vi "TestUplink.vi"(0 "RFSA Handle In":refnum<k15>="PXI1Slot5" caption="RFSA Handle in", 1 "UL Rx Span":i64=200000, 2 "SMU Handle In":refnum<k15> caption="SMU Handle in", 3 "UL Tx Payload (Hex)":string, 4 "UL Data Rate":i64=600, 5 "Resp Timeout (ms)":i32, 6 "FPGA Reference":refnum<k20>, 7 "error in (no error)":errorcluster, 8 "UL Freq Offset (Hz)":i64=1, 9 "UL Pwr Reduction (dB/2)":i8=-34, 10 "DxSupply":string, 11 "UL Tx Freq (Hz)":i64=1, 13 "UL Rx Timeout":i64=60, 14 "Enum":T1, 15 "UL Rx Central Freq":i64=902200000) -> (12 "Send UL OK":bool, 21 "Meas UL Rx Freq":i64, 23 "UL Rx Payload":string, 24 "Meas UL Idd":dbl, 27 "error out":errorcluster)   [LabVIEW 2018]
uses:
  Resources_Test/UART/ControlTestSlot.ctl
  <vilib>/Analysis/4window.llb/windowTd.ctl
  <vilib>/measure/maspectr.llb/FFT Power Spectrum and PSD for 1 Chan (CDB).vi
  <vilib>/measure/NI_MAPro.lvlib
  <vilib>/Analysis/NI_AALPro.lvlib
panel:
  out "Timeout Flag":bool
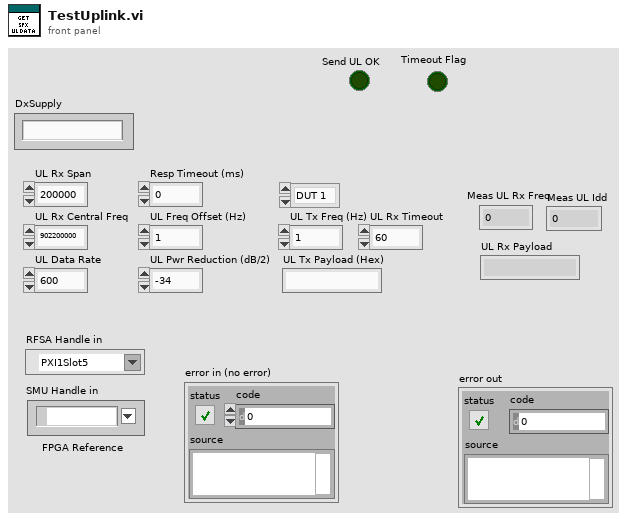
[diagram p1: front panel]
types:
  T1 = typedef "ControlTestSlot.ctl" = enum16{"DUT 1", "DUT 2"}
  T2 = cluster{"averaging mode":enum16{"No averaging", "Vector averaging", "RMS averaging", "Peak hold"}, "weighting mode":enum16{"Linear", "Exponential"}, "number of averages":u32}
  T3 = typedef "NI_AALPro.lvlib/windowTd.ctl" = u32
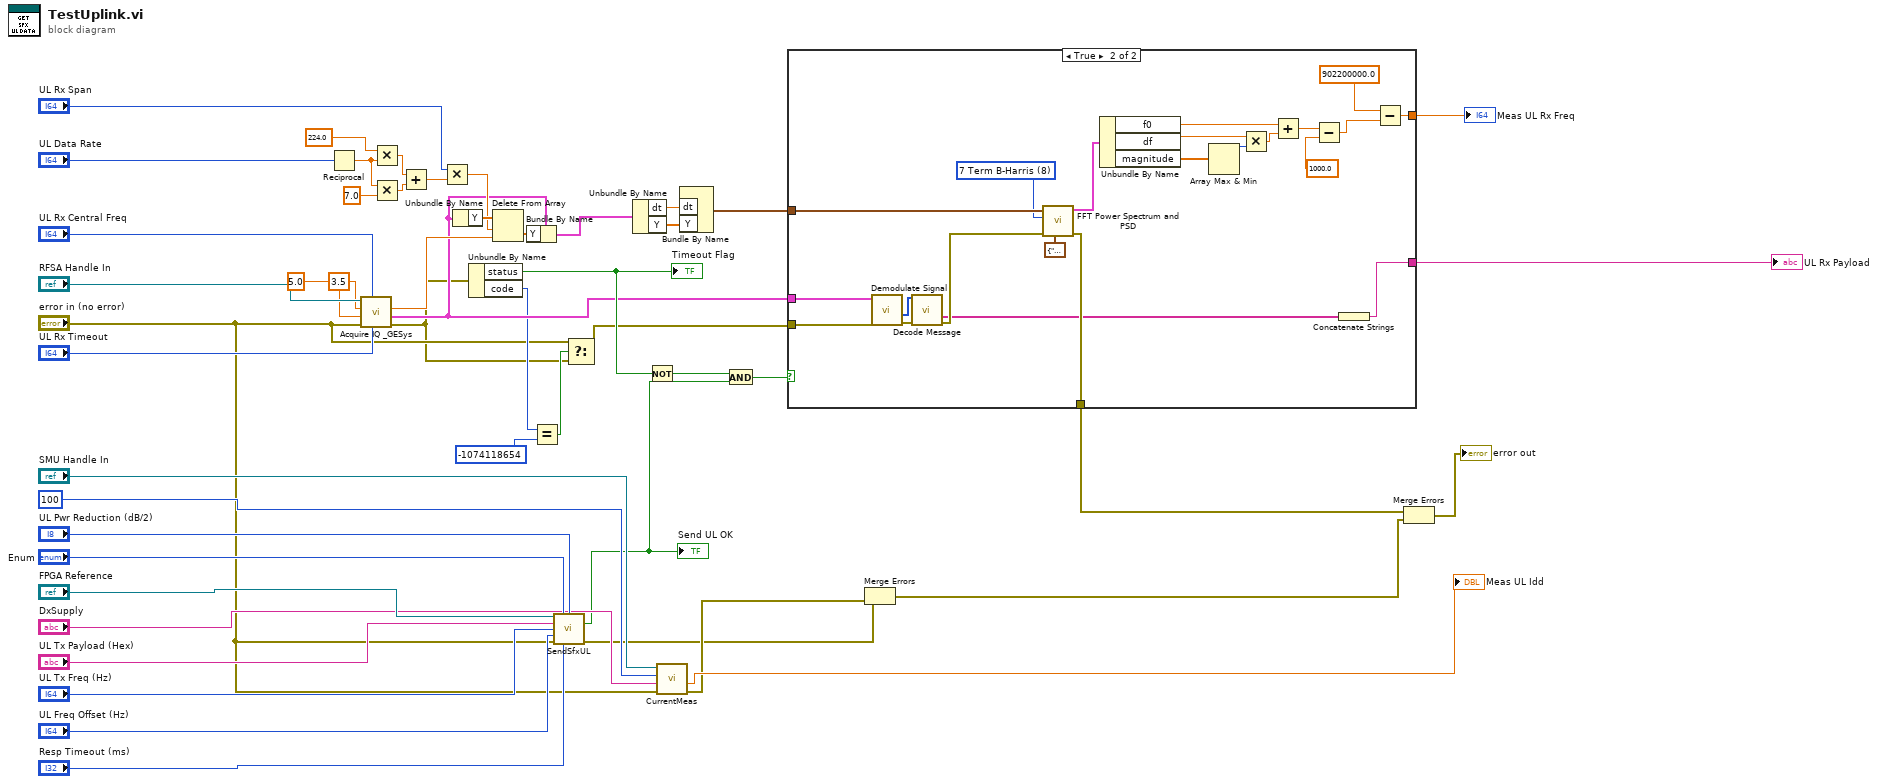
[diagram p0: block diagram]
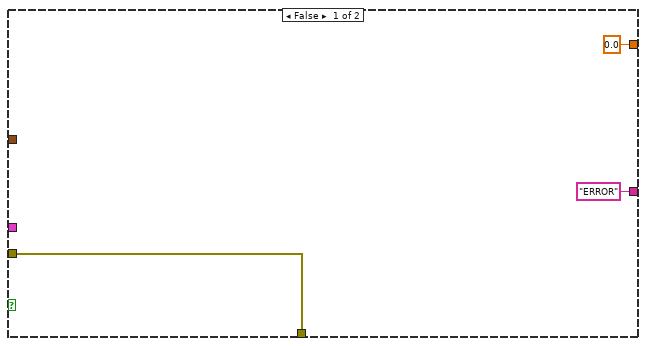
[diagram p2: hidden frame]
diagram:
  n1 = Reciprocal(x="UL Data Rate") -> (1/x=w27:dbl)
  n2 = call "Acquire IQ _GESys.vi"("timeout (10 sec)"="UL Rx Timeout", "Carrier Frequency (Hz)"="UL Rx Central Freq", "error in (no error)"="error in (no error)", "Reference Position (%)"=5.0, "Burst Length (sec)"=3.5, "instrument handle"="RFSA Handle In") -> ("error out"=w2:errorcluster, "IQ"=w8:cluster{"t0":dbl, "dt":dbl, "Y":cdb[]}, "Pre-Trigger"=w21:dbl)  [unwired: 2 in, 1 out]
  n3 = Multiply(x=224.0, y=w27) -> (x*y=w24:dbl)
  n4 = Multiply(x=w27, y=7.0) -> (x*y=w23:dbl)
  n5 = Add(x=w24, y=w23) -> (x+y=w25:dbl)
  n6 = Multiply(x="UL Rx Span", y=w25) -> (x*y=w22:dbl)
  n7 = Unbundle By Name(w8) -> ("Y"=w29:cdb[])
  n8 = Unbundle By Name(w2) -> ("status"=w15:bool, "code"=w6:i32)
  "Timeout Flag" <- w15
  n9 = Delete From Array(array=w29, length=w22, index=w21) -> (deleted portion=w20:cdb[])  [unwired: 1 out]
  n10 = Bundle By Name(cluster=w8, "Y"=w20) -> (w16:cluster{"t0":dbl, "dt":dbl, "Y":cdb[]})
  n11 = Equal?(x=w6, y=-1074118654) -> (x = y?=w4:bool)
  n12 = call "SendSfxUL.vi"("FPGA Reference"="FPGA Reference", "Enum"="Enum", "Pwr Reduction (dB/2)"="UL Pwr Reduction (dB/2)", "Tx Payload (Hex)"="UL Tx Payload (Hex)", "Tx Freq (Hz)"="UL Tx Freq (Hz)", "Freq Offset (Hz)"="UL Freq Offset (Hz)", "Error In"="error in (no error)", "Resp Timeout (ms)"="Resp Timeout (ms)") -> ("Send UL OK"=w13:bool, "Error Out"=w30:errorcluster)  [unwired: 6 in]
  "Send UL OK" <- w13
  n13 = Select(t="error in (no error)", s=w4, f=w2) -> (s? t:f=w1:errorcluster)
  n14 = Unbundle By Name(w16) -> ("dt"=w19:dbl, "Y"=w18:cdb[])
  n15 = Not(x=w15) -> (.not. x?=w14:bool)
  n16 = call "CurrentMeas.vi"("error in (no error)"="error in (no error)", "DxSupply"="DxSupply", "Measure Record Length"=100, "instrument handle"="SMU Handle In") -> ("error out"=w31:errorcluster, "Idd Peak"=→"Meas UL Idd":dbl)  [unwired: 4 in, 2 out]
  n17 = Bundle By Name("dt"=w19, "Y"=w18) -> (w17:waveform(cdb))  [unwired: 1 in]
  n18 = And(x=w14, y=w13) -> (x .and. y?=w9:bool)
  n19 = case shown="True" w9 {
    tunnel: [0.0 w75] -> w36
    tunnel: w17 -> [_ w74]
    tunnel: [w51 w61] -> w12
    tunnel: w1 -> [w51 w60]
    tunnel: w8 -> [_ w59]
    tunnel: ["ERROR" w54] -> w7
    frame False {
    }
    frame True {
      w66 = T3 8 items=["Rectangle"=0, "Hanning"=1, "Hamming"=2, "Blackman-Harris"=3, "Exact Blackman"=4, "Blackman"=5, "Flat Top"=6, "4 Term B-Harris "=7, "7 Term B-Harris"=8, "Low Sidelobe"=9, "Blackman Nuttall"=11, "Triangle"=30, "Bartlett-Hanning"=31, "Bohman"=32, "Parzen"=33, "Welch"=34, "Kaiser"=60, "Dolph-Chebyshev"=61, "Gaussian"=62] ("window")
      n20 = call "Demodulate Signal.vi"("error in (no error)"=w60, "Complex Waveform"=w59) -> ("error out"=w56:errorcluster, "Output bit stream"=w57:i8[])  [unwired: 6 in, 2 out]
      n21 = call "Decode Message.vi"("Bit Stream"=w57, "error in"=w56) -> ("Payload"=w55:string[], "error out"=w58:errorcluster)  [unwired: 8 in, 4 out]
      n22 = call-poly <vilib>:"FFT Power Spectrum and PSD.vi"("averaging parameters"=T2 {"averaging mode"=enum."Peak hold", "weighting mode"=enum."Exponential", "number of averages"=8}, "error in (no error)"=w58, "window"=w66, "time signal"=w74) -> ("error out"=w61:errorcluster, "Power Spectrum / PSD"=w73:cluster{"f0":dbl, "df":dbl, "magnitude":dbl[]})  [unwired: 4 in, 2 out]
      n23 = Unbundle By Name(w73) -> ("f0"=w71:dbl, "df"=w69:dbl, "magnitude"=w72:dbl[])
      n24 = Array Max & Min(array=w72) -> (max index (indices)=w68:i32)  [unwired: 3 out]
      n25 = Multiply(x=w69, y=w68) -> (x*y=w70:dbl)
      n26 = Add(x=w71, y=w70) -> (x+y=w64:dbl)
      n27 = Subtract(x=w64, y=1000.0) -> (x-y=w63:dbl)
      n28 = Concatenate Strings(w55) -> (w54:string)
      n29 = Subtract(x=902200000.0, y=w63) -> (x-y=w75:dbl)
    }
  }
  "Meas UL Rx Freq" <- w36
  "UL Rx Payload" <- w7
  n30 = Merge Errors(w30, w31) -> (w11:errorcluster)
  n31 = Merge Errors(w12, w11) -> (→"error out":errorcluster)
